vi "Warning.vi"(8 "error in (no error)":errorcluster, 9 "Source":string, 10 "Message":string, 11 "RQMHLogger in":refnum<class "Logger.lvclass">) -> (0 "error out":errorcluster, 3 "RQMHLogger out":refnum<class "Logger.lvclass">)   [LabVIEW 2024, in "Logger.lvclass"]
uses:
  Logger.lvclass
  Logger.lvclass/Logger.ctl
  Record/LogRecord.lvclass/LogRecord.ctl
  HandleHolder/HandleHolder.lvclass/HandleHolder.ctl
  Record/LogRecord.lvclass
  LogHandle/Interface/LoggingHandle.lvclass
  Shared/Level.ctl
  Shared/LoggerShared.lvlib
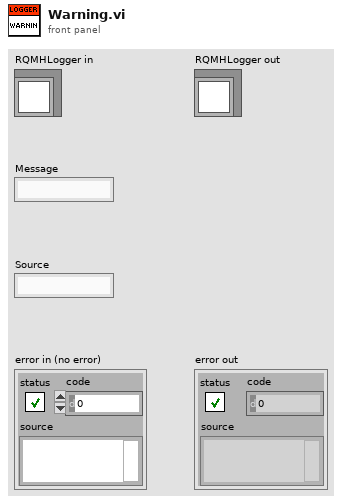
[diagram p1: front panel]
types:
  T1 = typedef "LoggerShared.lvlib/Level.ctl" = enum16{"DEBUG", "INFO", "WARNING", "ERROR", "CRITICAL"}
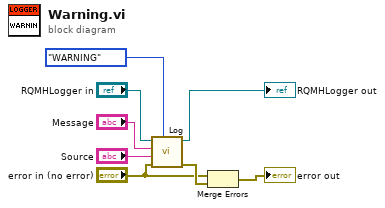
[diagram p0: block diagram]
diagram:
  n1 = call "Log.vi"("Level"=Level."WARNING", "Error to log"="error in (no error)", "Source"="Source", "Message"="Message", "RQMHLogger in"="RQMHLogger in") -> ("Errors"=w3:errorcluster[], "RQMHLogger out"=→"RQMHLogger out":refnum<class "Logger.lvclass">)  [unwired: 5 in]
  n2 = Merge Errors("error in (no error)", w3) -> (→"error out":errorcluster)
